vi "Read Parameter FIle.vi"(8 "error in":errorcluster, 11 "path in":path) -> (0 "error out":errorcluster, 2 "Parameter map":T1(c390), 3 "path out":path)   [LabVIEW 2020, in "Ballard 1553 System Explorer.lvlib"]
uses:
  Ballard 1553 System Explorer.lvlib
  89334f65-b8d8-493c-8c0a-5e818c4493ce.vi
  <vilib>/JDP Science/JSONtext/JSON text to Variant.vi
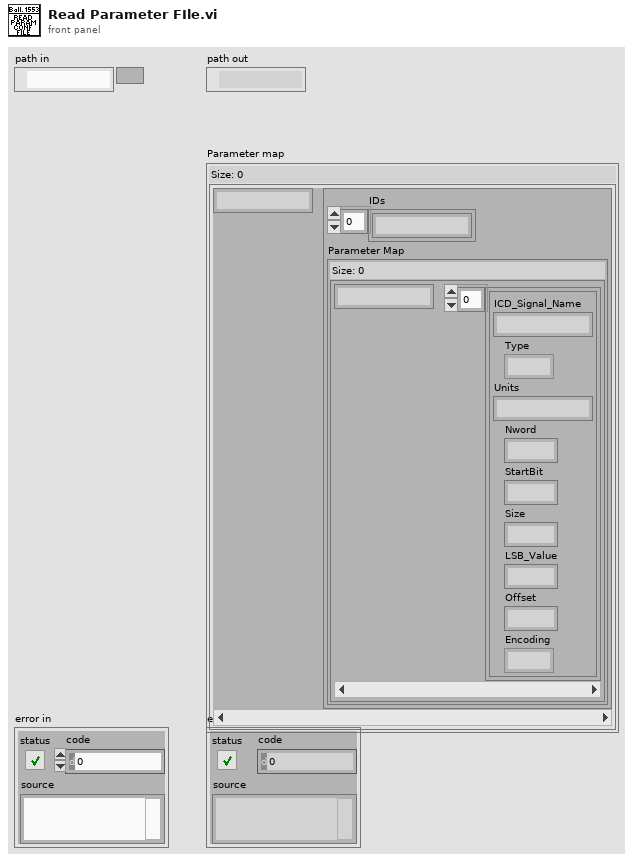
[diagram p1: front panel]
types:
  T1 = map{string, cluster{"IDs":string[], "Parameter Map":map{string, cluster{"ICD_Signal_Name":string, "Type":enum16{"Opaque", "Enum", "Float", "Integer", "Bcd", "Bool"}, "Units":string, "Nword":i32, "StartBit":i32, "Size":i32, "LSB_Value":i32, "Offset":i32, "Encoding":enum16{"None", "2-complement", "Unsigned"}}[]}}}
  T2 = cluster{"BusName":string, "Messages":cluster{"Id":string, "Signals":cluster{"ICD_Signal_Name":string, "Type":enum16{"Opaque", "Enum", "Float", "Integer", "Bcd", "Bool"}, "Units":string, "Nword":i32, "StartBit":i32, "Size":i32, "LSB_Value":i32, "Offset":i32, "Encoding":enum16{"None", "2-complement", "Unsigned"}}[]}[]}[]
  T3 = cluster{"IDs":string[], "Parameter Map":map{string, cluster{"ICD_Signal_Name":string, "Type":enum16{"Opaque", "Enum", "Float", "Integer", "Bcd", "Bool"}, "Units":string, "Nword":i32, "StartBit":i32, "Size":i32, "LSB_Value":i32, "Offset":i32, "Encoding":enum16{"None", "2-complement", "Unsigned"}}[]}}
  T4 = map{string, cluster{"ICD_Signal_Name":string, "Type":enum16{"Opaque", "Enum", "Float", "Integer", "Bcd", "Bool"}, "Units":string, "Nword":i32, "StartBit":i32, "Size":i32, "LSB_Value":i32, "Offset":i32, "Encoding":enum16{"None", "2-complement", "Unsigned"}}[]}
  T5 = cluster{"Id":string, "Signals":cluster{"ICD_Signal_Name":string, "Type":enum16{"Opaque", "Enum", "Float", "Integer", "Bcd", "Bool"}, "Units":string, "Nword":i32, "StartBit":i32, "Size":i32, "LSB_Value":i32, "Offset":i32, "Encoding":enum16{"None", "2-complement", "Unsigned"}}[]}[]
  T6 = cluster{"ICD_Signal_Name":string, "Type":enum16{"Opaque", "Enum", "Float", "Integer", "Bcd", "Bool"}, "Units":string, "Nword":i32, "StartBit":i32, "Size":i32, "LSB_Value":i32, "Offset":i32, "Encoding":enum16{"None", "2-complement", "Unsigned"}}[]
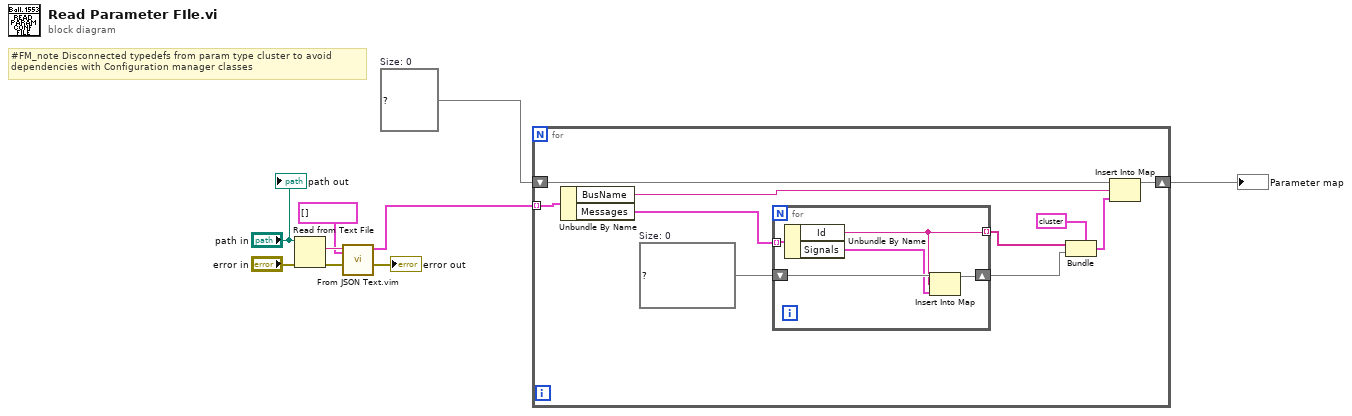
[diagram p0: block diagram]
diagram:
  w2 = T1 {}  # Size: 0
  # "#FM_note Disconnected typedefs from param type cluster to avoid\ndependencies with Configuration manager classes"
  n1 = Read from Text File(file (use dialog)="path in", error in="error in") -> (text=w8:string, error out=w9:errorcluster)  [unwired: 2 in, 2 out]
  n2 = call "From JSON Text.vim"("Data Type and Default Value"=T2 [], "error in (no error)"=w9, "JSON"=w8) -> ("error out"=→"error out":errorcluster, "Data out"=w5:T2)  [unwired: 7 in]
  n3 = for {
    shift-right: [w18] -> w1
    shift-left: w2 -> [w19]
    tunnel: w5 -> [w17] mode=indexing
    w14 = T4 {}  # Size: 0
    n4 = Unbundle By Name(w17) -> ("BusName"=w16:string, "Messages"=w15:T5)
    n5 = for {
      tunnel: w15 -> [w22] mode=indexing
      shift-right: [w23] -> w12
      shift-left: w14 -> [w24]
      tunnel: [w20] -> w13 mode=indexing
      n6 = Unbundle By Name(w22) -> ("Id"=w20:string, "Signals"=w21:T6)
      n7 = Insert Into Map(map in=w24, key=w20, value=w21) -> (map out=w23:T4)  [unwired: 2 out]
    }
    n8 = Bundle(cluster=T3 {"IDs"=[], "Parameter Map"={}}, "IDs"=w13, "Parameter Map"=w12) -> (w10:T3)
    n9 = Insert Into Map(map in=w19, key=w16, value=w10) -> (map out=w18:T1)  [unwired: 2 out]
  }
  "Parameter map" <- w1
  "path out" <- "path in"
